vi "Save Bitfile Settings.vi"(8 "error in (no error)":errorcluster, 9 "Bitfile Info":T2, 10 "Path":path, 11 "Device Ref in":T1 format="%.0x") -> (0 "error out":errorcluster, 3 "Device Ref out":T1 format="%.0x")   [LabVIEW 2014, in "SLSC configuration System Explorer.lvlib"]
uses:
  SLSC configuration System Explorer.lvlib
  Type Defs/SLSC Bitfile Info.ctl
  <vilib>/NI Veristand/Custom Device API/Custom Device Item Ref.ctl
  Shared/Constants.vi
  <vilib>/NI Veristand/Custom Device API/Set Item Property (String).vi
  <vilib>/NI Veristand/Custom Device API/Set Item Property (U16).vi
  <vilib>/NI Veristand/Custom Device API/Set Item Property (Dependent File).vi
  <vilib>/NI Veristand/Custom Device API/Custom Device API.lvlib
  Shared/SLSC configuration Shared.lvlib
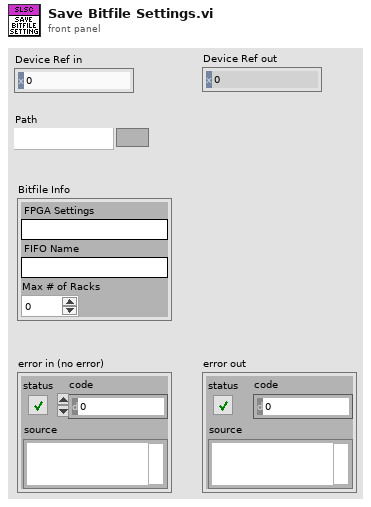
[diagram p1: front panel]
types:
  T1 = typedef "Custom Device API.lvlib/Custom Device Item Ref.ctl" = u64
  T2 = typedef "SLSC configuration System Explorer.lvlib/SLSC Bitfile Info.ctl" = cluster{"FPGA Settings":string, "FIFO Name":string, "Max # of Racks":u8}
  T3 = typedef "Custom Device API.lvlib/Dependent File Optional Info.ctl" = cluster{"Version":string, "RTDestination":path, "ForceDownload":bool, "SupportedTarget":string, "MD5":string}
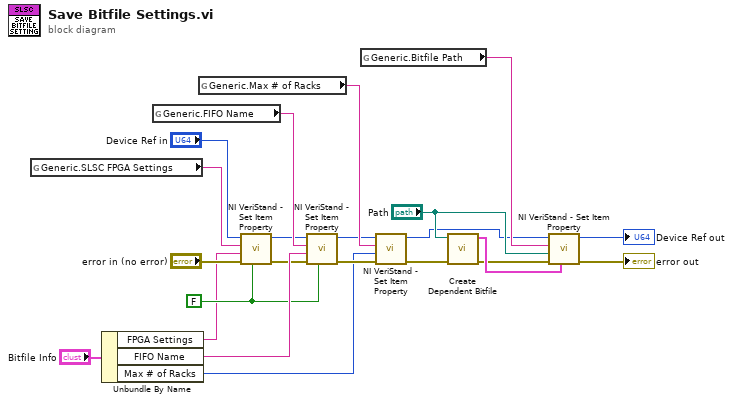
[diagram p0: block diagram]
diagram:
  w16 = FALSE ("Binary String (T)")
  n1 = global read "Constants.vi" "Generic.SLSC FPGA Settings"() -> (w11:string)
  n2 = Unbundle By Name("Bitfile Info") -> ("FPGA Settings"=w12:string, "FIFO Name"=w17:string, "Max # of Racks"=w1:u8)
  n3 = global read "Constants.vi" "Generic.FIFO Name"() -> (w15:string)
  n4 = global read "Constants.vi" "Generic.Max # of Racks"() -> (w6:string)
  n5 = call-poly <vilib>:"NI VeriStand - Set Item Property.vi"("Binary String (T)"=w16, "error in (no error)"="error in (no error)", "Value"=w12, "Property Name"=w11, "Item Ref in"="Device Ref in") -> ("error out"=w13:errorcluster, "Item Ref out"=w14:T1)  [unwired: 4 in, 1 out]
  n6 = call-poly <vilib>:"NI VeriStand - Set Item Property.vi"("Binary String (T)"=w16, "error in (no error)"=w13, "Value"=w17, "Property Name"=w15, "Item Ref in"=w14) -> ("error out"=w4:errorcluster, "Item Ref out"=w5:T1)  [unwired: 4 in, 1 out]
  n7 = global read "Constants.vi" "Generic.Bitfile Path"() -> (w7:string)
  n8 = call-poly <vilib>:"NI VeriStand - Set Item Property.vi"("error in (no error)"=w4, "Value"=w1, "Property Name"=w6, "Item Ref in"=w5) -> ("error out"=w3:errorcluster, "Item Ref out"=w2:T1)  [unwired: 5 in, 1 out]
  n9 = call "Create Dependent Bitfile.vi"("error in (no error)"=w3, "Path"="Path") -> ("error out"=w8:errorcluster, "OptionalInfo"=w9:T3)  [unwired: 8 in]
  n10 = call-poly <vilib>:"NI VeriStand - Set Item Property.vi"("OptionalInfo"=w9, "error in (no error)"=w8, "Path"="Path", "Property Name"=w7, "Item Ref in"=w2) -> ("error out"=→"error out":errorcluster, "Item Ref out"=→"Device Ref out":T1)  [unwired: 4 in, 1 out]
